vi "NT_LL_Read Integer.vi"(8 "error in (no error)":errorcluster, 10 "default value":i64, 11 "subscribeHandle":u32) -> (0 "error out":errorcluster, 2 "time":i64, 3 "value":i64)   [LabVIEW 2025]
uses:
  FRC_NetworkTablesLV.dll
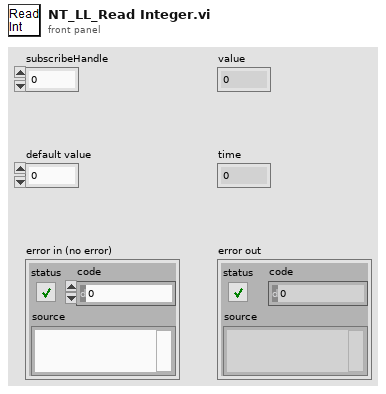
[diagram p1: front panel]
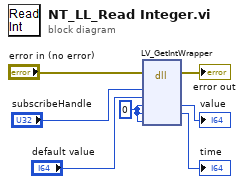
[diagram p0: block diagram]
diagram:
  w5 = 0
  n1 = dll-call lib="FRC_NetworkTablesLV.*" fn="LV_GetIntWrapper"(error in="error in (no error)", "subscribeHandle"="subscribeHandle", "default"="default value", "value"=w5, "time"=w5, "serverTime"=w5) -> (error out=→"error out":errorcluster, "value"=→"value":i64, "time"=→"time":i64)  [unwired: 6 in, 1 out]
